vi "Close.vi"(8 "error in (no error)":errorcluster, 11 "PacificPowerSource in":refnum<class "PacificPowerSource.lvclass">) -> (0 "error out":errorcluster, 3 "PacificPowerSource out":refnum<class "PacificPowerSource.lvclass">)   [LabVIEW 2018, in "AcPwrPlugins.lvlib" / "PacificPowerSource.lvclass"]
doc: "This VI closes the reference to the instrument."
uses:
  PacificPowerSource.lvclass
  C:/Users/ico/Documents/Projects/NistPluggableModules/AcPwr/AcPwrPlugins/AcPwrBaseClass/AcPwrBase.lvclass
  AcPwrBaseClass/AcPwrBase.lvclass/AcPwrBase.ctl
  AcPwrBaseClass/Accessors/Read BaseConfig.vi
  AcPwrBaseClass/Accessors/Write BaseConfig.vi
  <instrlib>/Pacific Power UPC Series/Pacific Power UPC Series.lvlib
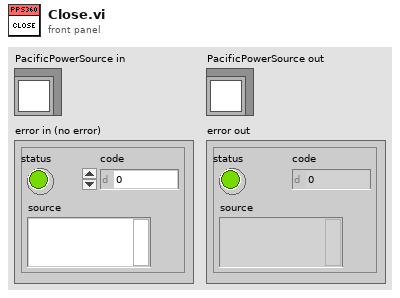
[diagram p1: front panel]
types:
  T1 = typedef "AcPwrPlugins.lvlib/AcPwrBase.lvclass/BaseConfig.ctl" = cluster{"Frequency":dbl, "FrequencyRange":dbl[], "Phases":T2[], "Name":string, "Chroma":T3, "NHRDC":T4, "PPS":T5}
  T2 = typedef "AcPwrPlugins.lvlib/AcPwrBase.lvclass/Phase.ctl" = cluster{"Name":string, "Enabled":bool, "VoltageLevel":dbl, "Handle":string, "VoltageRange":dbl[], "Connected":bool, "CurrentLimit":dbl, "Waveform":string}
  T3 = typedef "AcPwrPlugins.lvlib/ChromaAcLoad.lvclass/DeviceProperties.ctl" = cluster{"Configuration Mode":enum16{"Constant Voltage (DC)", "Constant Power (DC)", "Constant Power (AC)", "Constant Current (DC)", "Constant Current (AC)", "Constant Resistance (DC)", "Constant Resistance (AC)", "Rectified Mode (DC)", "Inrush (AC)", "RLC CP (AC)", "RLC (AC)"}, "Phases":cluster{"Handle":string, "Name":string, "Phase Select":i32, "Instrument Options":string, "id query (T)":bool, "reset device (T)":bool, "Load Short Circuited":bool, "Line Synchronization":bool, "Load Current (A/Arms)":dbl, "Load Voltage (V/Vrms)":dbl, "Load Power (W)":dbl, "Load Resistance (Ohms)":dbl, "Load Current Peak Limit (A)":dbl, "Load Current Limit (A/Arms)":dbl, "Load Power Limit (W)":dbl, "Synch Frequency (Hz)":dbl, "Priority":enum16{"CF Only", "PF Only", "Both (CF)", "Both (PF)"}, "Crest Factor":dbl, "Power Factor":dbl, "Slew Rate":cluster{"Rise Slew Rate (A/ms)":i32, "Fall Slew Rate (A/ms)":i32}, "LC/RLC Mode":cluster{"Capacitance (uF)":i32, "Inductance (uH)":i32, "Series Resistance (Ohm)":dbl, "Parallel Resistance (Ohm)":dbl}, "Timing":cluster{"TimingOn":enum16{""}, "Hours":u32, "Minutes":u32, "Seconds":dbl, "CutoffVoltage":dbl}, "Connected":bool}[]}
  T4 = typedef "AcPwrPlugins.lvlib/NHRDCPower.lvclass/Device(s)Settings.ctl" = cluster{"Handle":string, "Name":string, "id query (Yes)":bool, "reset device (Yes)":bool, "Connected":bool, "Voltage Range (V)":dbl[], "Timing":cluster{"TimingOn":enum16{""}, "Hours":u32, "Minutes":u32, "Seconds":dbl, "CutoffVoltage":dbl}, "Initial Battery Detect Voltage (0)":sgl, "SafetySettings":cluster{"SetWatchDog":bool, "Voltage (V)":sgl, "Current (A)":sgl, "Power (W)":sgl, "Voltage Delay (s)":sgl, "Current Delay (s)":sgl, "Power Delay (s)":sgl}, "Options String":string, "Aperture Time (s)":sgl, "operating state (Off)":i32, "OutputSettings":cluster{"Voltage (V)":sgl, "Current (A)":sgl, "Resistance (Ohms)":sgl, "Power (W)":sgl, "Enable Voltage":bool, "Enable Current":bool, "Enable Resistance":bool, "Enable Power":bool, "Delay After (s)":sgl, "Wait Value (V, A, W)":sgl, "Enable Wait":bool, "Wait on Value":i32}[], "SlewRate":cluster{"Set Voltage Rate V/S":sgl, "Set Current Rate A/S":sgl, "Set Resistance Rate R/S":sgl, "Set Power Rate W/S":sgl}}[]
  T5 = typedef "AcPwrPlugins.lvlib/PacificPowerSource.lvclass/DeviceSettings.ctl" = cluster{"Handle":string, "Connected":bool, "Clear Device (F)":bool, "btnIdQuery":bool, "btnReset":bool, "Program #":cluster{"Phase B (Degrees)":i32, "Waveform A (1: Sine)":i32, "Voltage Level (Va)":dbl, "Program Number (0)":i32, "Voltage Level (Vb) ":dbl, "Form (3: Three)":u16, "Coupling  (0: Direct)":u16, "Frequency (45Hz)":dbl, "Current Limit (40A)":dbl, "Phase C (Degrees)":i32, "Voltage Level (Vc)":dbl, "Waveform B (1: Sine)":i32, "Waveform C (1: Sine)":i32}[], "Impedance Parameters (off, 0.00)":cluster{"State":bool, "Impedance":dbl}, "Transient Execution (F)":bool, "OutputEnabled":bool, "Source Range":cluster{"Frequency Minimum (45 Hz)":dbl, "Frequency Maximum (1200 Hz)":dbl, "Voltage Maximum (V)":dbl, "Voltage Minimum (V)":dbl, "Range Control (0: Auto)":u16, "Initial Voltage (0V)":u16, "Frequency Range (600Hz)":u16}, "Port Type":enum16{"GPIB", "Serial"}}[]
  T6 = cluster{"Handle":string, "Connected":bool, "Clear Device (F)":bool, "btnIdQuery":bool, "btnReset":bool, "Program #":cluster{"Phase B (Degrees)":i32, "Waveform A (1: Sine)":i32, "Voltage Level (Va)":dbl, "Program Number (0)":i32, "Voltage Level (Vb) ":dbl, "Form (3: Three)":u16, "Coupling  (0: Direct)":u16, "Frequency (45Hz)":dbl, "Current Limit (40A)":dbl, "Phase C (Degrees)":i32, "Voltage Level (Vc)":dbl, "Waveform B (1: Sine)":i32, "Waveform C (1: Sine)":i32}[], "Impedance Parameters (off, 0.00)":cluster{"State":bool, "Impedance":dbl}, "Transient Execution (F)":bool, "OutputEnabled":bool, "Source Range":cluster{"Frequency Minimum (45 Hz)":dbl, "Frequency Maximum (1200 Hz)":dbl, "Voltage Maximum (V)":dbl, "Voltage Minimum (V)":dbl, "Range Control (0: Auto)":u16, "Initial Voltage (0V)":u16, "Frequency Range (600Hz)":u16}, "Port Type":enum16{"GPIB", "Serial"}}
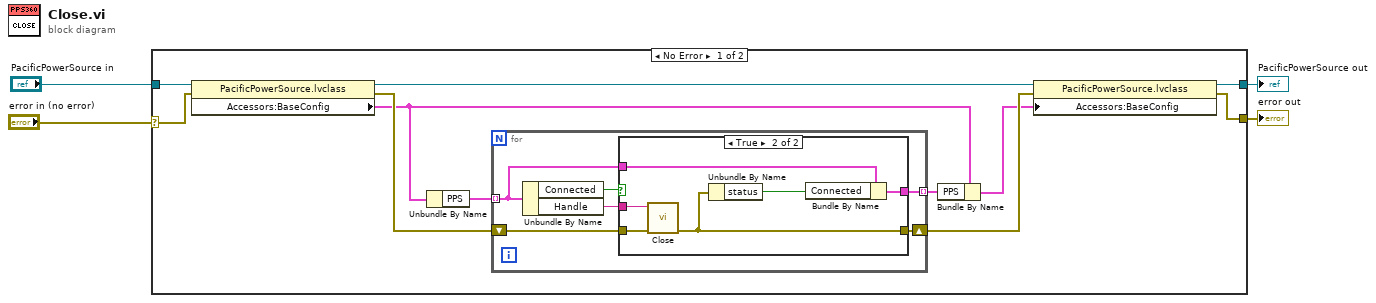
[diagram p0: block diagram]
diagram:
  n1 = case shown="No Error" "error in (no error)" {
    selector: "error in (no error)" -> [w14 w31]
    tunnel: [w11 w31] -> w4
    tunnel: [w9 w30] -> w3
    tunnel: "PacificPowerSource in" -> [w15 w30]
    frame No Error {
      n2 = property class="PacificPowerSource.lvclass"(reference=w15, error in=w14) -> (reference out=w10:refnum<class "PacificPowerSource.lvclass">, error out=w13:errorcluster, "Accessors:BaseConfig"=w7:T1)
      n3 = Unbundle By Name(w7) -> ("PPS"=w8:T5)
      n4 = for {
        shift-right: [w20] -> w12
        shift-left: w13 -> [w21]
        tunnel: w8 -> [w17] mode=indexing
        tunnel: [w16] -> w6 mode=indexing
        n5 = Unbundle By Name(w17) -> ("Connected"=w18:bool, "Handle"=w19:string)
        n6 = case shown="True" w18 {
          tunnel: w21 -> [w23 w29]
          tunnel: [w23 w25] -> w20
          tunnel: w19 -> [_ w28]
          tunnel: w17 -> [w22 w27]
          tunnel: [w22 w26] -> w16
          frame False {
          }
          frame True {
            n7 = call <instrlib>:"Close.vi"("error in (no error)"=w29, "VISA resource name"=w28) -> ("error out"=w25:errorcluster)  [unwired: 9 in]
            n8 = Unbundle By Name(w25) -> ("status"=w24:bool)
            n9 = Bundle By Name(cluster=w27, "Connected"=w24) -> (w26:T6)
          }
        }
      }
      n10 = Bundle By Name(cluster=w7, "PPS"=w6) -> (w5:T1)
      n11 = property class="PacificPowerSource.lvclass"(reference=w10, error in=w12, "Accessors:BaseConfig"=w5) -> (reference out=w9:refnum<class "PacificPowerSource.lvclass">, error out=w11:errorcluster)
    }
    frame Error {
    }
  }
  "error out" <- w4
  "PacificPowerSource out" <- w3
